vi "FindProxyClassObject.vi"(0 "remote class ref":refnum<class "G#Object.lvclass">, 5 "error in (no error)":errorcluster) -> (14 "proxy class ref":refnum<class "G#RemoteProxy.lvclass">, 17 "found":bool, 19 "error out":errorcluster)   [LabVIEW 2017, in "G#RemoteProxy.lvclass"]
doc: "Finds the proxy class object."
uses:
  G#RemoteProxy.lvclass
  G#Object/G#Object.lvclass
  G#DebugServer/G#DebugServer.lvclass
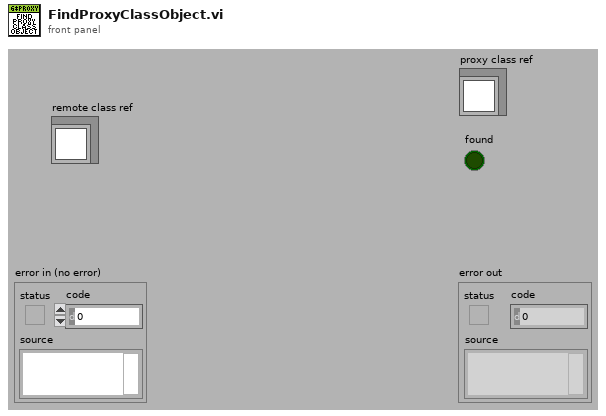
[diagram p1: front panel]
types:
  T1 = typedef "G#RemoteProxy.lvclass/ClassAttributesProxy.ctl" = cluster{"NoActiveProject":bool, "FullClassNames":string[], "FullClassPaths":path[], "RemoteRefs":refnum<class "G#Object.lvclass">[], "ProxyRefs":refnum<class "G#RemoteProxy.lvclass">[], "RemoteClassName":string[], "ProxyClassRefs":refnum<class "G#RemoteProxy.lvclass">[]}
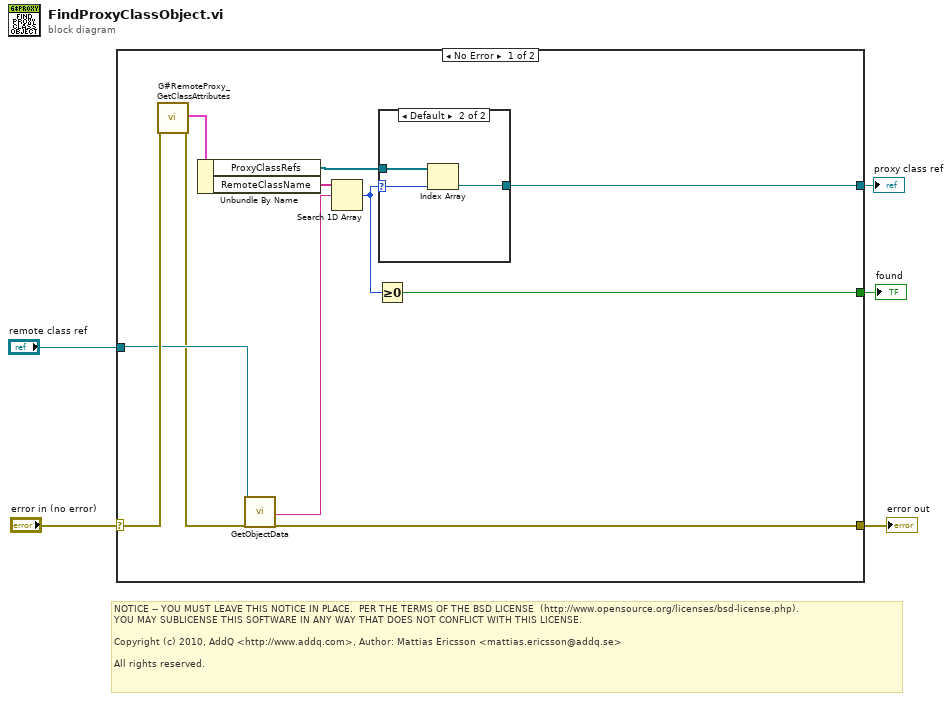
[diagram p0: block diagram]
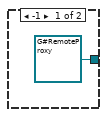
[diagram p2: hidden frame]
diagram:
  # "NOTICE -- YOU MUST LEAVE THIS NOTICE IN PLACE.  PER THE TERMS OF THE BSD LICENSE  (http://www.opensource.org/licenses/bsd-license.php).\nYOU MAY SUBLICENSE THIS SOFTWARE IN ANY WAY THAT DOES NOT CONFLICT WITH THIS LICENSE.\n\nCopyright (c) 2010, AddQ <http://www.addq.com>, Author: Mattias Ericsson <mattias.ericsson@addq.se>\n\nAll rights reserved."
  n1 = case shown="No Error" "error in (no error)" {
    selector: "error in (no error)" -> [w16 w21]
    tunnel: [w7 w21] -> w4
    tunnel: "remote class ref" -> [w9 _]
    tunnel: [w12 _] -> w2
    tunnel: [w10 _] -> w1
    frame No Error {
      n2 = call "G#RemoteProxy_GetClassAttributes.vi"("error in (no error)"=w16) -> ("class attributes"=w15:T1, "error out"=w8:errorcluster)  [unwired: 15 in, 2 out]
      n3 = Unbundle By Name(w15) -> ("ProxyClassRefs"=w13:refnum<class "G#RemoteProxy.lvclass">[], "RemoteClassName"=w14:string[])
      n4 = call "GetObjectData.vi"("remote ref"=w9, "error in (no error)"=w8) -> ("FullClassName"=w6:string, "error out"=w7:errorcluster)  [unwired: 13 in, 3 out]
      n5 = Search 1D Array(1D array=w14, element=w6) -> (index of element=w11:i32)  [unwired: 1 in]
      n6 = Greater Or Equal To 0?(x=w11) -> (x >= 0?=w10:bool)
      n7 = case shown="Default" w11 {
        selector: w11 -> [_ w19]
        tunnel: w13 -> [_ w20]
        tunnel: [refnum<class "G#RemoteProxy.lvclass"> refnum ("G#RemoteProxy.lvclass") w18] -> w12
        frame -1 {
        }
        frame Default {
          n8 = Index Array(array=w20, index=w19) -> (element=w18:refnum<class "G#RemoteProxy.lvclass">)
        }
      }
    }
    frame Error {
    }
  }
  "error out" <- w4
  "proxy class ref" <- w2
  "found" <- w1
